vi "ExampleMenu.vi"() -> ()   [LabVIEW 2013]
panel:
  in  "Menu Cluster":T1
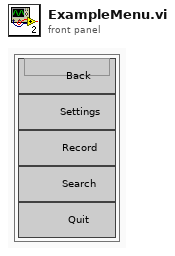
[diagram p1: front panel]
types:
  T1 = cluster{"Settings Button":bool, "Search Button":bool, "Record Button":bool, "Quit Button":bool, "Back Button":bool}
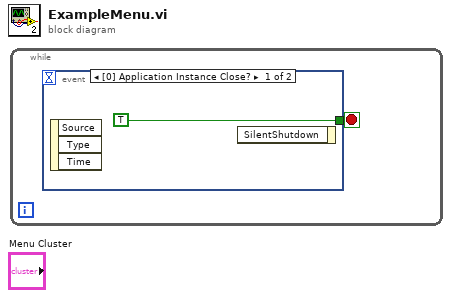
[diagram p0: block diagram]
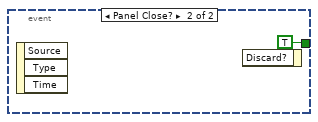
[diagram p2: hidden frame]
diagram:
  n1 = while {
    stop <- w1 stop-if-true
    n2 = event shown="[0] Application Instance Close?" {
      selector: _ -> [_ _]
      dyn-events: _ -> [_ _]
      timeout: _ -> [_ _]
      tunnel: [TRUE TRUE] -> w1
      event Application Instance Close? {
        n3 = event-data() -> ()  [unwired: 1 in, 3 out]
        n4 = event-data() -> ()  [unwired: 2 in, 1 out]
      }
      event Panel Close? {
        n5 = event-data() -> ()  [unwired: 1 in, 3 out]
        n6 = event-data() -> ()  [unwired: 2 in, 1 out]
      }
    }
  }
